vi "PIDController_New.vi"(9 "Kd":dbl, 10 "Ki":dbl, 11 "Kp":dbl) -> (3 "PID_CONTROLLER":T1={"Kp"=0.0, "Ki"=0.0, "Kd"=0.0, "Period"=0.0, "Max_Integral"=0.0, "Min_Integral"=0.0, "Max_Input"=0.0, "Min_Input"=0.0, "Continuous"=FALSE, "PositionError"=0.0, "VelocityError"=0.0, "PrevError"=0.0, "TotalError"=0.0, "PositionTolerance"=0.0, "VelocityTolerance"=0.0, "SetPoint"=0.0, "Kf"=0.0, "Prev_Deriv"=0.0, "Prev_Deriv 2"=0.0, "DerivativeFilter"=FALSE, "Min_Output"=-9.99e+35, "Max_Output"=9.9e+35, "Prev_F_P"=0.0, "Prev_F_P_2"=0.0, "AntiWindupActive"=FALSE, "Measurement"=0.0} {"Measurement" format="%16_6e"; "Prev_F_P_2" format="%16_6e"; "Prev_F_P" format="%16_6e"; "Max_Output" format="%16_6e"; "Min_Output" format="%16_6e"; "Prev_Deriv 2" format="%16_6e"; "Prev_Deriv" format="%16_6e"; "Kf" format="%16_6e"; "SetPoint" format="%16_6e"; "VelocityTolerance" format="%16_6e"; "PositionTolerance" format="%16_6e"; "TotalError" format="%16_6e"; "PrevError" format="%16_6e"; "VelocityError" format="%16_6e"; "PositionError" format="%16_6e"; "Min_Input" format="%16_6e"; "Max_Input" format="%16_6e"; "Min_Integral" format="%16_6e"; "Max_Integral" format="%16_6e"; "Period" format="%16_6e"; "Kd" format="%16_6e"; "Ki" format="%16_6e"; "Kp" format="%16_6e"})   [LabVIEW 2019, in "Trajectory_Library.lvlib"]
doc: "Allocates a PIDController data cluster with the given constants for Kp, Ki, and Kd and a default period of 0.02 seconds.\n\nImplements a PID control loop. This data structure also can be used with the \"Advanced\" PID calculation subVIs.\n \nInputs:\n - Kp -- The proportional coefficient.\n - Ki -- The integral coefficient.\n - Kd -- The derivative coefficient.\n\nOutputs:\n - PID_Controller -- Initialized PID_Controller data cluster"
uses:
  Trajectory_Library.lvlib
  TypeDef/PID_CONTROLLER.ctl
  <vilib>/Rock Robotics/SystemInterfaces/NetworkCommunication/NetComm_UsageReport_report.vi
  Util_LibraryGlobals.vi
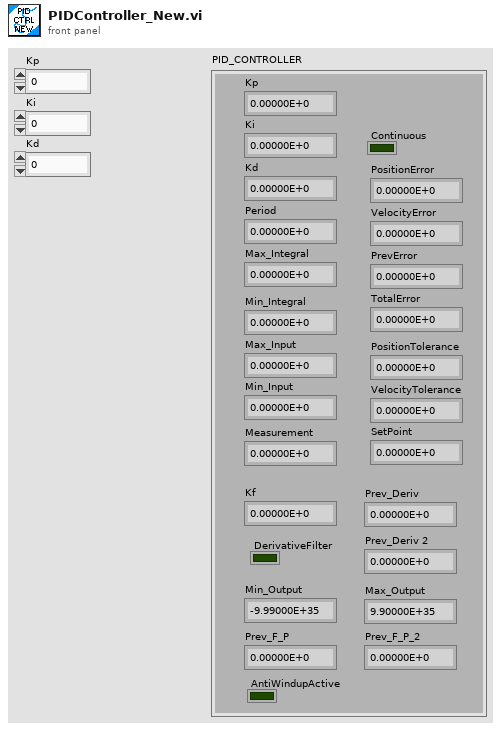
[diagram p1: front panel]
types:
  T1 = typedef "Trajectory_Library.lvlib/PID_CONTROLLER.ctl" = cluster{"Kp":dbl, "Ki":dbl, "Kd":dbl, "Period":dbl, "Max_Integral":dbl, "Min_Integral":dbl, "Max_Input":dbl, "Min_Input":dbl, "Continuous":bool, "PositionError":dbl, "VelocityError":dbl, "PrevError":dbl, "TotalError":dbl, "PositionTolerance":dbl, "VelocityTolerance":dbl, "SetPoint":dbl, "Kf":dbl, "Prev_Deriv":dbl, "Prev_Deriv 2":dbl, "DerivativeFilter":bool, "Min_Output":dbl, "Max_Output":dbl, "Prev_F_P":dbl, "Prev_F_P_2":dbl, "AntiWindupActive":bool, "Measurement":dbl}
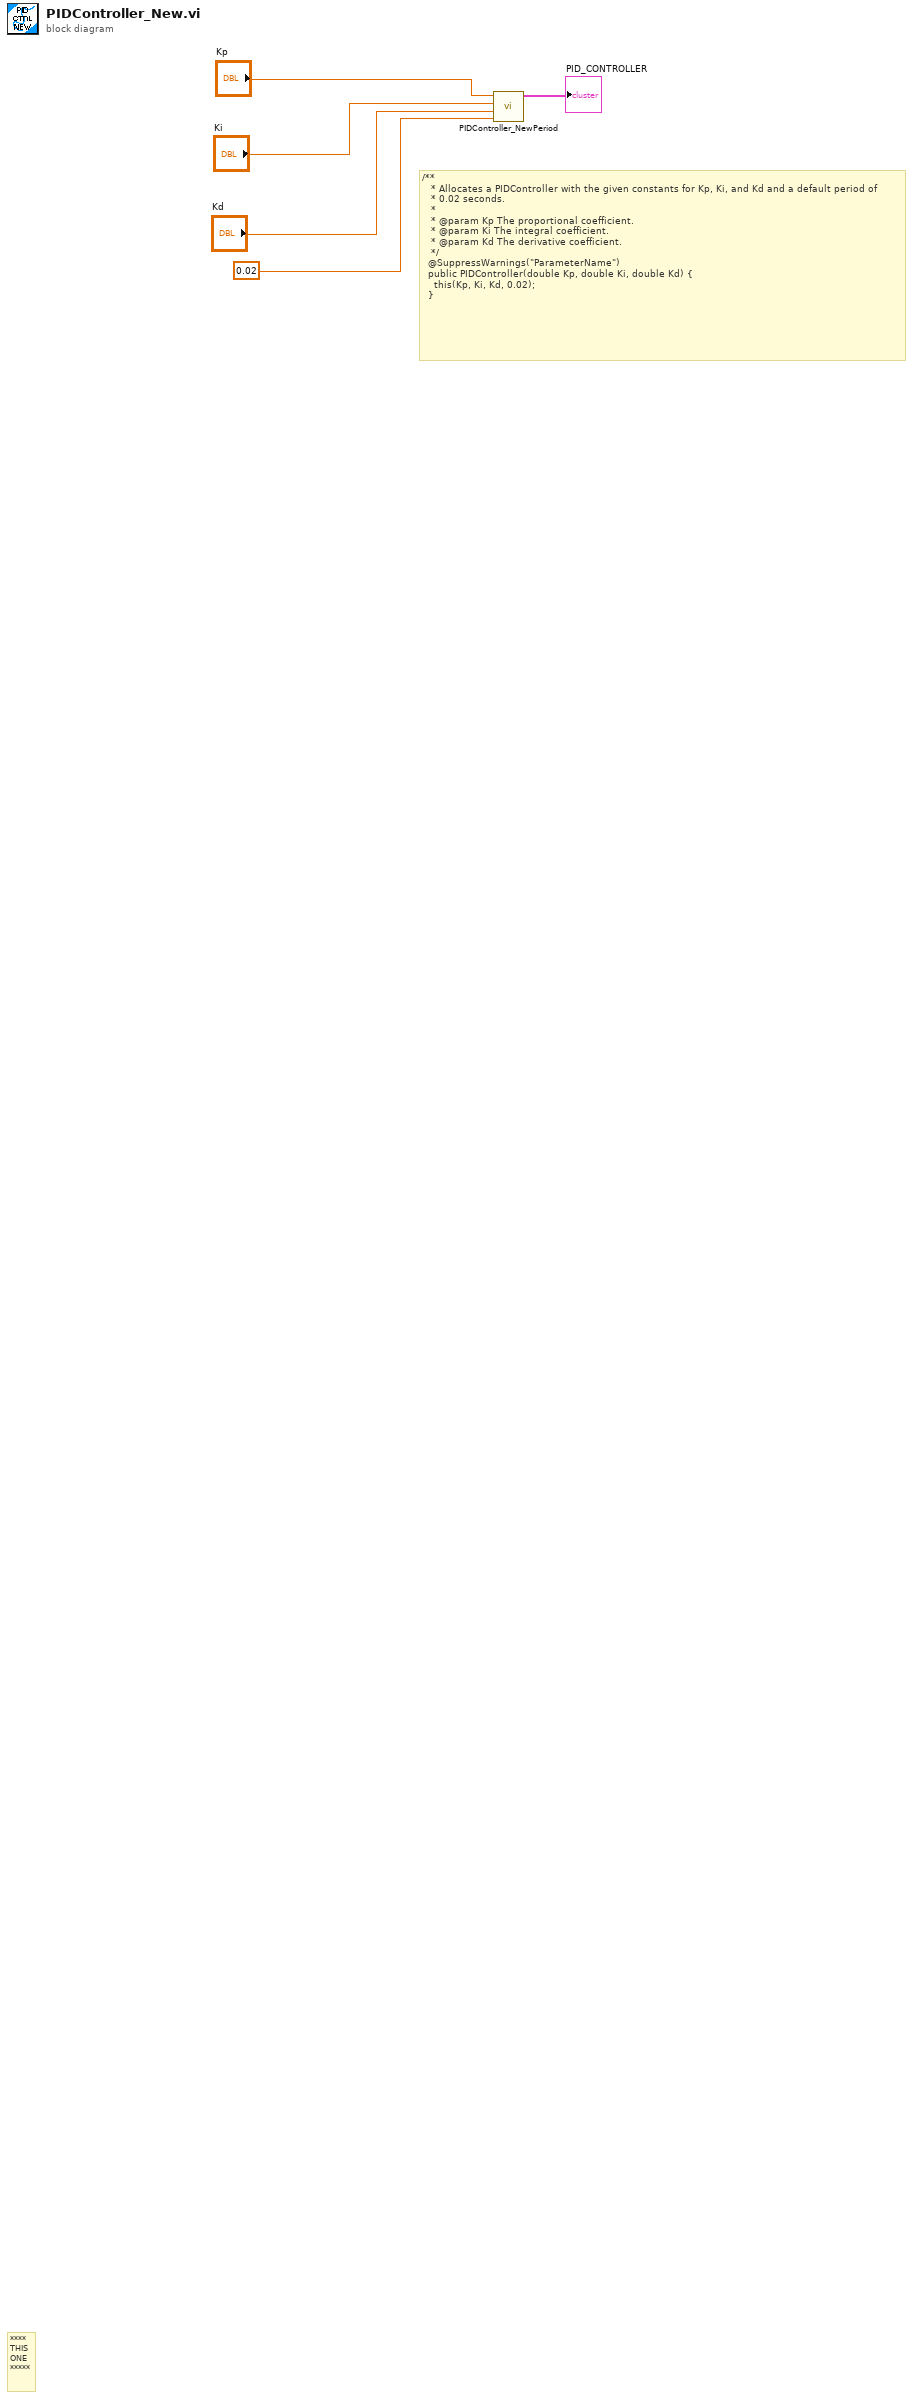
[diagram p0: block diagram]
diagram:
  # "/**\n   * Allocates a PIDController with the given constants for Kp, Ki, and Kd and a default period of\n   * 0.02 seconds.\n   *\n   * @param Kp The proportional coefficient.\n   * @param Ki The integral coefficient.\n   * @param Kd The derivative coefficient.\n   */\n  @SuppressWarnings(\"ParameterName\")\n  public PIDController(double Kp, double Ki, double Kd) {\n    this(Kp, Ki, Kd, 0.02);\n  }"
  # "****\nTHIS\nONE\n*****"
  n1 = call "PIDController_NewPeriod.vi"("Period"=0.02, "Kd"="Kd", "Ki"="Ki", "Kp"="Kp") -> ("PID_CONTROLLER"=→"PID_CONTROLLER":T1)  [unwired: 7 in]
